vi "二型板测试报告存储.vi"(11 "试验时间":timestamp) -> ()   [LabVIEW 2010]
uses:
  全局量/试验配置信息.vi
  全局量/自动测试结果.vi
panel:
  in  "序号":i32
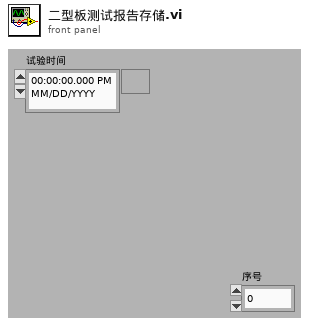
[diagram p1: front panel]
types:
  T1 = cluster{"position (Excel)":cluster{"row":i32, "column":i32}, "name (Excel)":string, "bookmark (Word)":string}
  T2 = cluster{"报告编号":string, "控制板编号":string, "控制板类型":string, "测试人员":string, "测试地点":string, string, u64, "spreadsheet string":string, "spreadsheet string":string, "spreadsheet string":string, "spreadsheet string":string}
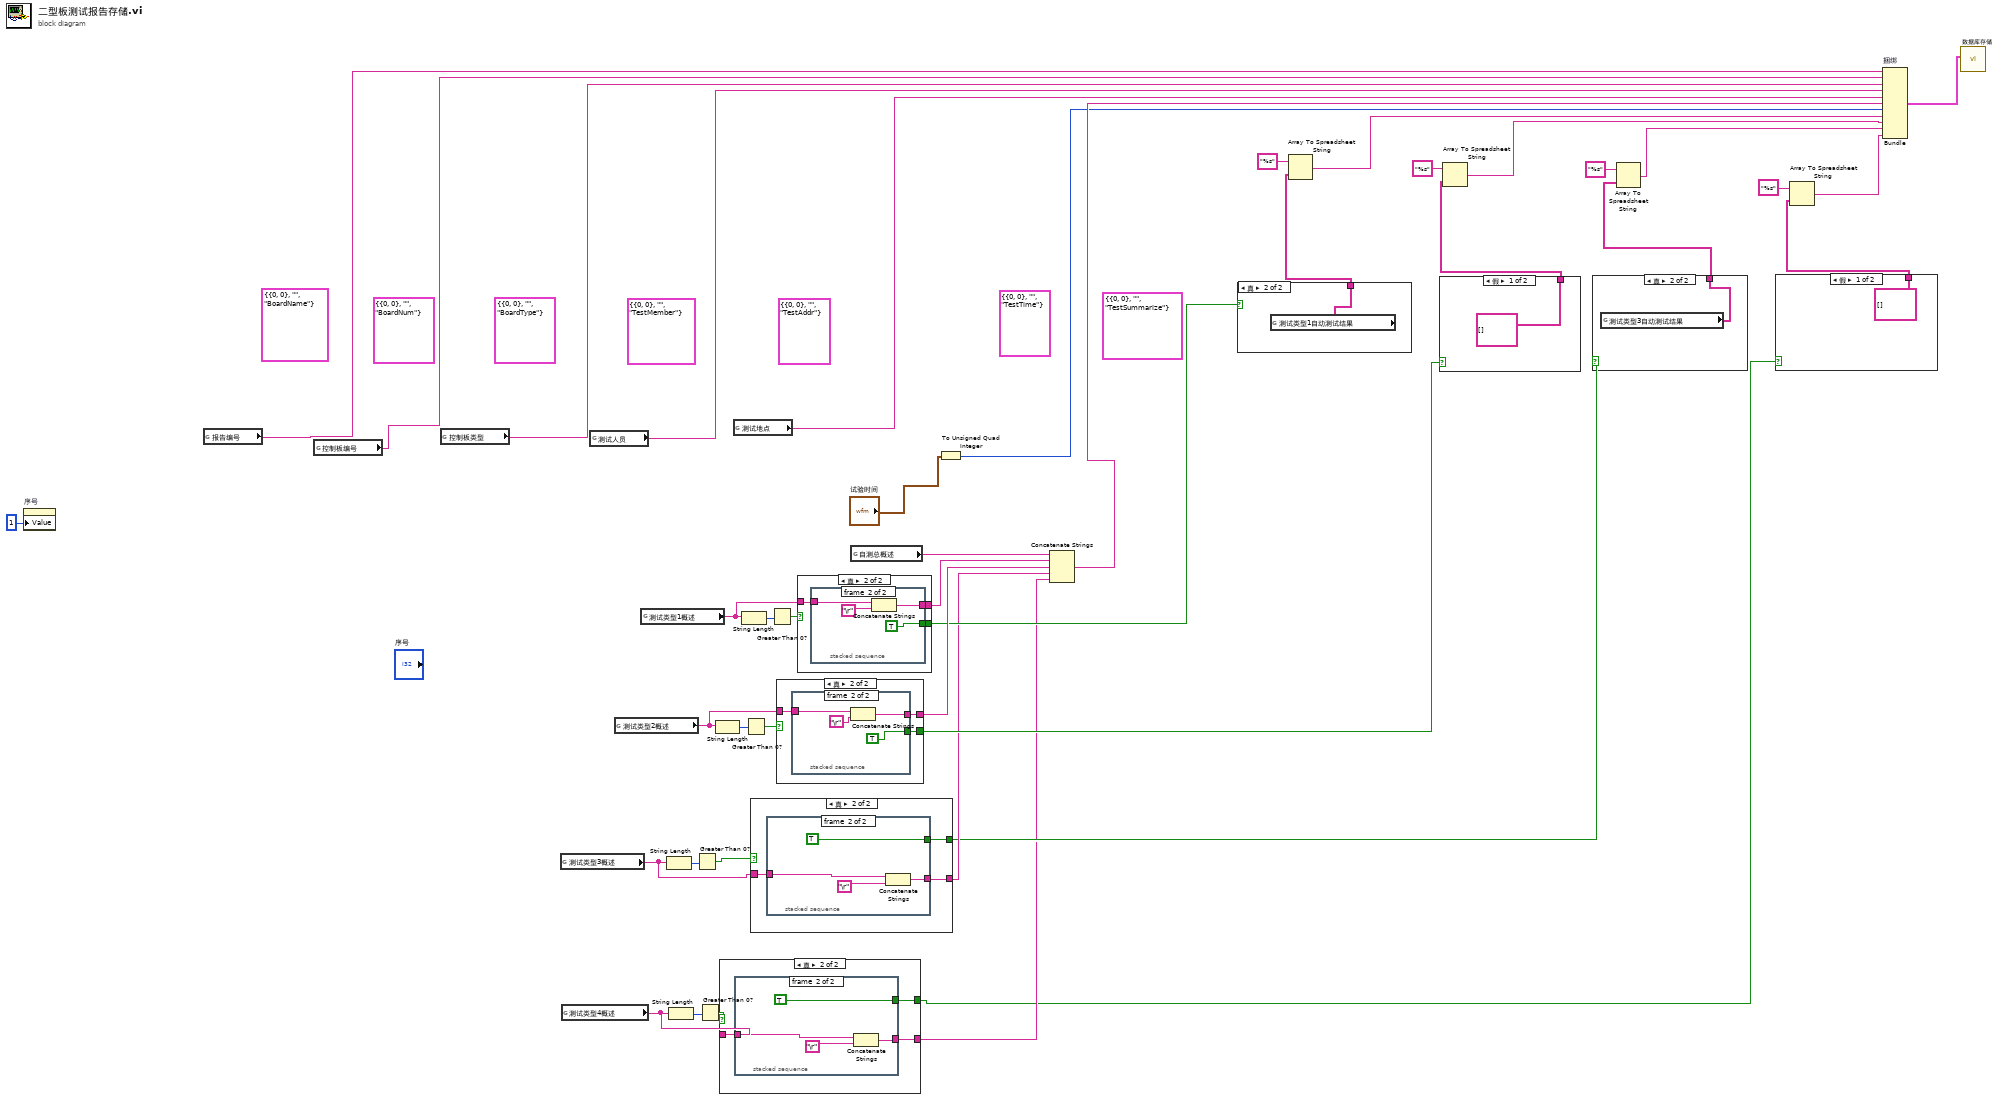
[diagram p0: block diagram]
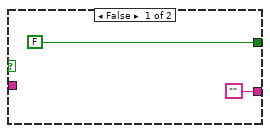
[diagram p2: hidden frame]
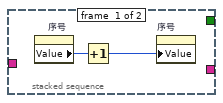
[diagram p3: hidden frame]
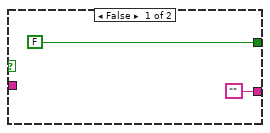
[diagram p4: hidden frame]
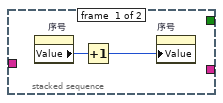
[diagram p5: hidden frame]
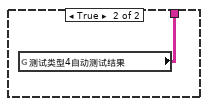
[diagram p6: hidden frame]
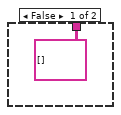
[diagram p7: hidden frame]
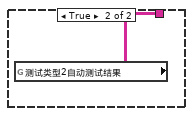
[diagram p8: hidden frame]
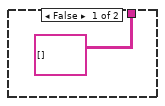
[diagram p9: hidden frame]
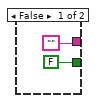
[diagram p10: hidden frame]
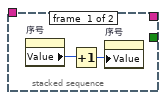
[diagram p11: hidden frame]
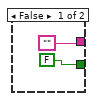
[diagram p12: hidden frame]
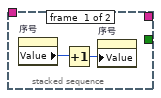
[diagram p13: hidden frame]
diagram:
  (unwired) T1 {"position (Excel)"={"row"=0, "column"=0}, "name (Excel)"="", "bookmark (Word)"="TestSummarize"} ("MS Office parameters")
  (unwired) T1 {"position (Excel)"={"row"=0, "column"=0}, "name (Excel)"="", "bookmark (Word)"="TestAddr"} ("MS Office parameters")
  (unwired) T1 {"position (Excel)"={"row"=0, "column"=0}, "name (Excel)"="", "bookmark (Word)"="TestMember"} ("MS Office parameters")
  (unwired) T1 {"position (Excel)"={"row"=0, "column"=0}, "name (Excel)"="", "bookmark (Word)"="BoardType"} ("MS Office parameters")
  (unwired) T1 {"position (Excel)"={"row"=0, "column"=0}, "name (Excel)"="", "bookmark (Word)"="BoardNum"} ("MS Office parameters")
  (unwired) T1 {"position (Excel)"={"row"=0, "column"=0}, "name (Excel)"="", "bookmark (Word)"="TestTime"} ("MS Office parameters")
  (unwired) T1 {"position (Excel)"={"row"=0, "column"=0}, "name (Excel)"="", "bookmark (Word)"="BoardName"} ("MS Office parameters")
  n1 = property on="序号" class="DigNum (严格)"("Value"=1 ("序号")) -> ()  [unwired: 2 in, 2 out]
  n2 = global read "试验配置信息.vi" "报告编号"() -> (w30:string)
  n3 = global read "试验配置信息.vi" "控制板编号"() -> (w29:string)
  n4 = global read "试验配置信息.vi" "控制板类型"() -> (w28:string)
  n5 = global read "自动测试结果.vi" "测试类型3概述"() -> (w6:string)
  n6 = global read "自动测试结果.vi" "测试类型4概述"() -> (w5:string)
  n7 = global read "试验配置信息.vi" "测试人员"() -> (w27:string)
  n8 = global read "自动测试结果.vi" "测试类型2概述"() -> (w40:string)
  n9 = global read "自动测试结果.vi" "测试类型1概述"() -> (w41:string)
  n10 = String Length(string=w6) -> (length=w10:i32)
  n11 = String Length(string=w5) -> (length=w3:i32)
  n12 = Greater Than 0?(x=w10) -> (x > 0?=w7:bool)
  n13 = Greater Than 0?(x=w3) -> (x > 0?=w4:bool)
  n14 = String Length(string=w40) -> (length=w38:i32)
  n15 = case shown="真" w4 {
    tunnel: ["" w47] -> w2
    tunnel: w5 -> [_ w48]
    tunnel: [FALSE w46] -> w1
    frame False {
    }
    frame True {
      n16 = stacked-sequence {
        tunnel: w48 -> [_ w54]
        tunnel: [_ w53] -> w47
        tunnel: [_ TRUE] -> w46
        frame #0 {
          n17 = property on="序号" class="DigNum (严格)"() -> ("Value"=w50:i32)  [unwired: 2 in, 2 out]
          n18 = Increment(x=w50) -> (x+1=w49:i32)
          n19 = property on="序号" class="DigNum (严格)"("Value"=w49) -> ()  [unwired: 2 in, 2 out]
        }
        frame #1 {
          n20 = Concatenate Strings(w54, "\r") -> (w53:string)
        }
      }
    }
  }
  n21 = global read "试验配置信息.vi" "测试地点"() -> (w26:string)
  n22 = String Length(string=w41) -> (length=w43:i32)
  n23 = Greater Than 0?(x=w38) -> (x > 0?=w39:bool)
  n24 = case shown="真" w7 {
    tunnel: ["" w58] -> w9
    tunnel: w6 -> [_ w59]
    tunnel: [FALSE w57] -> w8
    frame False {
    }
    frame True {
      n25 = stacked-sequence {
        tunnel: w59 -> [_ w65]
        tunnel: [_ w64] -> w58
        tunnel: [_ TRUE] -> w57
        frame #0 {
          n26 = property on="序号" class="DigNum (严格)"() -> ("Value"=w61:i32)  [unwired: 2 in, 2 out]
          n27 = Increment(x=w61) -> (x+1=w60:i32)
          n28 = property on="序号" class="DigNum (严格)"("Value"=w60) -> ()  [unwired: 2 in, 2 out]
        }
        frame #1 {
          n29 = Concatenate Strings(w65, "\r") -> (w64:string)
        }
      }
    }
  }
  n30 = Greater Than 0?(x=w43) -> (x > 0?=w42:bool)
  n31 = case shown="真" w39 {
    tunnel: w40 -> [_ w70]
    tunnel: ["" w69] -> w35
    tunnel: [FALSE w68] -> w32
    frame False {
    }
    frame True {
      n32 = stacked-sequence {
        tunnel: w70 -> [_ w76]
        tunnel: [_ w74] -> w69
        tunnel: [_ TRUE] -> w68
        frame #0 {
          n33 = property on="序号" class="DigNum (严格)"() -> ("Value"=w72:i32)  [unwired: 2 in, 2 out]
          n34 = Increment(x=w72) -> (x+1=w71:i32)
          n35 = property on="序号" class="DigNum (严格)"("Value"=w71) -> ()  [unwired: 2 in, 2 out]
        }
        frame #1 {
          n36 = Concatenate Strings(w76, "\r") -> (w74:string)
        }
      }
    }
  }
  n37 = case shown="真" w42 {
    tunnel: w41 -> [_ w81]
    tunnel: ["" w80] -> w36
    tunnel: [FALSE w79] -> w33
    frame False {
    }
    frame True {
      n38 = stacked-sequence {
        tunnel: w81 -> [_ w87]
        tunnel: [_ w85] -> w80
        tunnel: [_ TRUE] -> w79
        frame #0 {
          n39 = property on="序号" class="DigNum (严格)"() -> ("Value"=w82:i32)  [unwired: 2 in, 2 out]
          n40 = Increment(x=w82) -> (x+1=w83:i32)
          n41 = property on="序号" class="DigNum (严格)"("Value"=w83) -> ()  [unwired: 2 in, 2 out]
        }
        frame #1 {
          n42 = Concatenate Strings(w87, "\r") -> (w85:string)
        }
      }
    }
  }
  n43 = global read "自动测试结果.vi" "自测总概述"() -> (w37:string)
  n44 = To Unsigned Quad Integer(1:"试验时间") -> (0:w24:u64)
  n45 = Concatenate Strings(w37, w36, w35, w9, w2) -> (w25:string)
  n46 = case shown="真" w33 {
    tunnel: [string[][] [] ("DI自动测试结果") w89] -> w22
    frame False {
    }
    frame True {
      n47 = global read "自动测试结果.vi" "测试类型1自动测试结果"() -> (w89:string[][])
    }
  }
  n48 = Array To Spreadsheet String(array=w22, 3:"%s" ("格式字符串")) -> (spreadsheet string=w21:string)  [unwired: 1 in]
  n49 = case shown="假" w32 {
    tunnel: [string[][] [] ("DO自动测试结果") w91] -> w19
    frame False {
    }
    frame True {
      n50 = global read "自动测试结果.vi" "测试类型2自动测试结果"() -> (w91:string[][])
    }
  }
  n51 = Array To Spreadsheet String(array=w19, 3:"%s" ("格式字符串")) -> (spreadsheet string=w18:string)  [unwired: 1 in]
  n52 = case shown="真" w8 {
    tunnel: [string[][] [] ("AI自动测试结果") w93] -> w16
    frame False {
    }
    frame True {
      n53 = global read "自动测试结果.vi" "测试类型3自动测试结果"() -> (w93:string[][])
    }
  }
  n54 = Array To Spreadsheet String(array=w16, 3:"%s" ("格式字符串")) -> (spreadsheet string=w15:string)  [unwired: 1 in]
  n55 = case shown="假" w1 {
    tunnel: [string[][] [] ("总线通信自测结果") w95] -> w13
    frame False {
    }
    frame True {
      n56 = global read "自动测试结果.vi" "测试类型4自动测试结果"() -> (w95:string[][])
    }
  }
  n57 = Array To Spreadsheet String(array=w13, 3:"%s" ("格式字符串")) -> (spreadsheet string=w12:string)  [unwired: 1 in]
  n58 = Bundle "捆绑"("报告编号"=w30, "控制板编号"=w29, "控制板类型"=w28, "测试人员"=w27, "测试地点"=w26, w25, w24, "spreadsheet string"=w21, "spreadsheet string"=w18, "spreadsheet string"=w15, "spreadsheet string"=w12) -> (w11:T2)  [unwired: 1 in]
  n59 = call "数据库存储.vi"("输出簇 2"=w11) -> ()  [unwired: 10 in]
